vi "Get Position.vi"(8 "error in (no error)":errorcluster, 10 "Axis":i32, 11 ".NET Refnum in":refnum<k24>) -> (0 "error out":errorcluster, 2 "position":dbl, 3 ".NET Refnum out":refnum<k24>)   [LabVIEW 2020, in "ESP301-Driver.lvlib"]
uses:
  ESP301-Driver.lvlib
  Newport.ESP301.CommandInterface
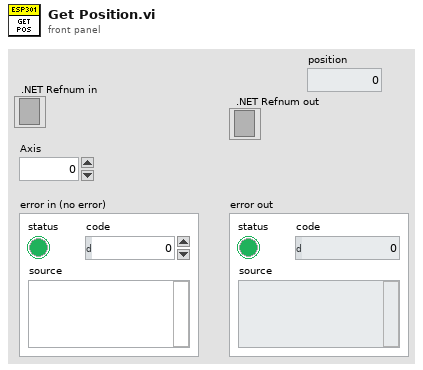
[diagram p1: front panel]
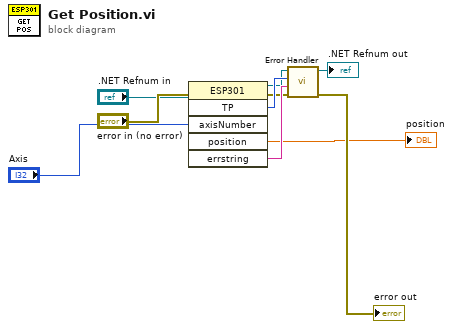
[diagram p0: block diagram]
diagram:
  n1 = invoke class="ESP301" method="TP"(reference=".NET Refnum in", error in="error in (no error)", "axisNumber"="Axis") -> (reference out=w8:refnum<k24>, error out=w4:errorcluster, "TP"=w9:i32, "position"=→"position":dbl, "errstring"=w10:string)  [unwired: 3 in, 1 out]
  n2 = call "Error Handler.vi"("error in (no error)"=w4, "Message"=w10, "Error Code"=w9, ".NET Refnum in"=w8) -> ("error out"=→"error out":errorcluster, ".NET Refnum out"=→".NET Refnum out":refnum<k24>)  [unwired: 6 in]
